vi "Overflow Protection.vi"(8 "error in (no error)":errorcluster, 9 "Display After":ext, 10 "Display Before":ext) -> (0 "error out":errorcluster, 2 "Display Output":ext)   [LabVIEW 2013]
doc: "This VI protects the Calculator against overflow, it will not allow numbers greater than 1E+15.\n\nAuthor: Erik Johnson, National Instruments"
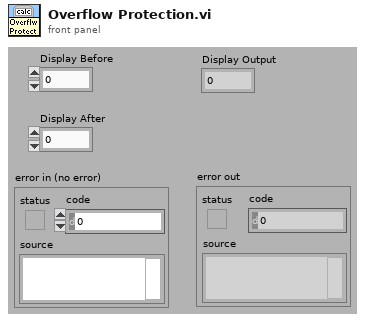
[diagram p1: front panel]
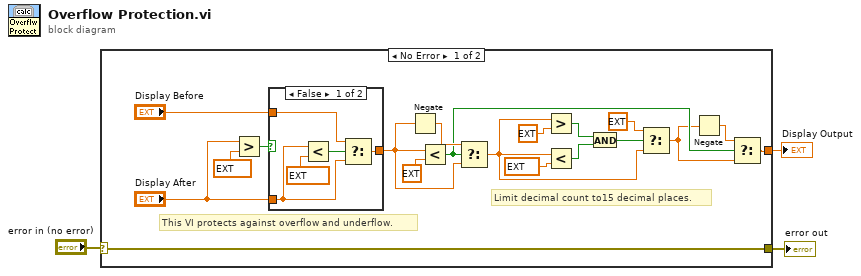
[diagram p0: block diagram]
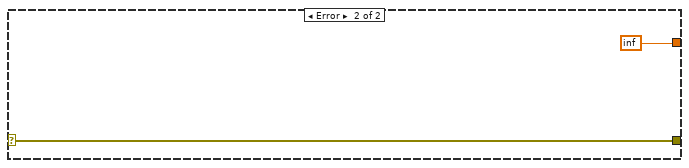
[diagram p3: hidden frame]
diagram:
  n1 = case shown="No Error" "error in (no error)" {
    selector: "error in (no error)" -> [w20 w30]
    tunnel: [w9 inf] -> w3
    tunnel: [w20 w30] -> w1
    frame No Error {
      # "Limit decimal count to15 decimal places."
      # "This VI protects against overflow and underflow."
      n2 = Greater?(x="Display After", y=ext 999999999999999.0) -> (0:w4:bool)
      n3 = case shown="False" w4 {
        tunnel: "Display After" -> [w23 _]
        tunnel: [w25 w28] -> w11
        tunnel: "Display Before" -> [w24 w28]
        frame False {
          n4 = Less?(x=w23, y=ext -1000000000000000.0) -> (x < y?=w26:bool)
          n5 = Select(t=w24, s=w26, f=w23) -> (s? t:f=w25:ext)
        }
        frame True {
        }
      }
      n6 = Negate(x=w11) -> (-x=w12:ext)
      n7 = Less?(x=w11, y=ext 0.0) -> (x < y?=w8:bool)
      n8 = Select(t=w12, s=w8, f=w11) -> (s? t:f=w10:ext)
      n9 = Greater?(x=w10, y=ext 0.0) -> (0:w17:bool)
      n10 = Less?(x=w10, y=ext 1e-15) -> (x < y?=w18:bool)
      n11 = And(x=w17, y=w18) -> (x .and. y?=w16:bool)
      n12 = Select(t=ext 0.0, s=w16, f=w10) -> (s? t:f=w7:ext)
      n13 = Negate(x=w7) -> (-x=w6:ext)
      n14 = Select(t=w6, s=w8, f=w7) -> (s? t:f=w9:ext)
    }
    frame Error {
    }
  }
  "Display Output" <- w3
  "error out" <- w1
